vi "Configure Harmonic.vi"(0 "VISA resource name":refnum<visa-resource-name>, 1 "Enable Harmonic (F:Disable)":bool, 2 "Phase (0 Degree)":dbl, 5 "Output Channel (1: Channel 1)":i32(ring)=1 items=["Channel 1"=1, "Channel 2"=2], 7 "Order (2)":i32=2, 9 "Harmonic Type (0: Even)":i32(ring) items=["Even", "Odd", "All"], 11 "error in (no error)":errorcluster, 12 "Amplitude (1 Vpp)":dbl=1.0) -> (4 "VISA resource name out":refnum<visa-resource-name>, 15 "error out":errorcluster)   [LabVIEW 2015, in "SDG X Series.lvlib"]
doc: "Configures and enables harmonic output."
uses:
  <instrlib>/SDG X Series/SDG X Series.lvlib
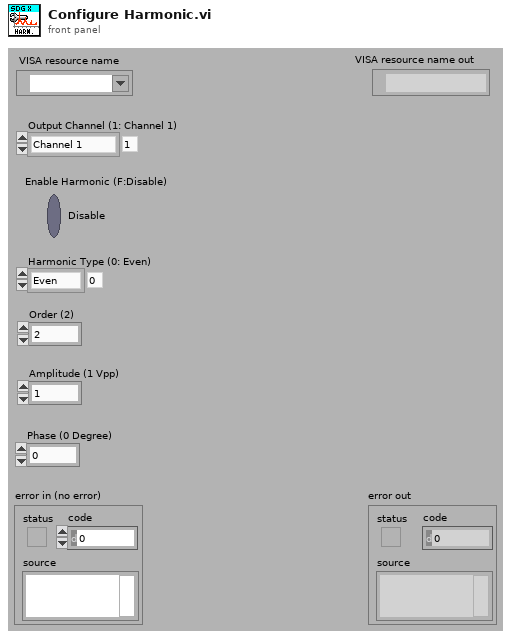
[diagram p1: front panel]
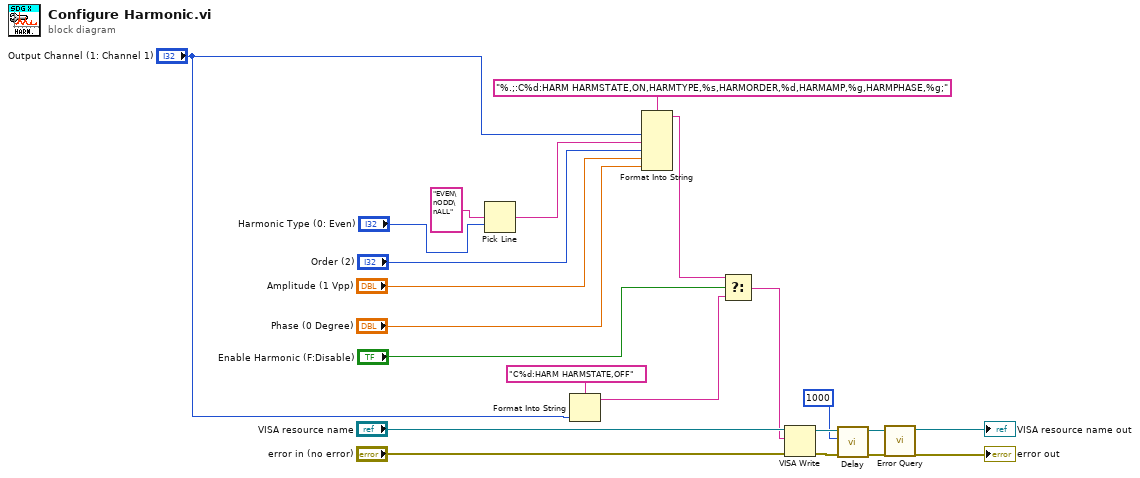
[diagram p0: block diagram]
diagram:
  n1 = Pick Line(multi-line string="EVEN\nODD\nALL", line index="Harmonic Type (0: Even)") -> (output string=w16:string)  [unwired: 1 out]
  n2 = Format Into String(format string="C%d:HARM HARMSTATE,OFF", "Output Channel (1: Channel 1)") -> (resulting string=w7:string)  [unwired: 2 in, 1 out]
  n3 = Format Into String(format string="%.;:C%d:HARM HARMSTATE,ON,HARMTYPE,%s,HARMORDER,%d,HARMAMP,%g,HARMPHASE,%g;", "Output Channel (1: Channel 1)", w16, "Order (2)", "Amplitude (1 Vpp)", "Phase (0 Degree)") -> (resulting string=w11:string)  [unwired: 2 in, 1 out]
  n4 = Select(t=w11, s="Enable Harmonic (F:Disable)", f=w7) -> (s? t:f=w10:string)
  n5 = VISA Write(VISA resource name="VISA resource name", write buffer=w10, error in (no error)="error in (no error)") -> (VISA resource name out=w3:refnum<visa-resource-name>, error out=w2:errorcluster)  [unwired: 1 out]
  n6 = call <instrlib>:"Delay.vi"("error in (no error)"=w2, "Delay Time (10)"=u32 1000, "VISA resource name"=w3) -> ("error out"=w5:errorcluster, "VISA resource name out"=w4:refnum<visa-resource-name>)  [unwired: 7 in]
  n7 = call <instrlib>:"Error Query.vi"("error in (no error)"=w5, "VISA resource name"=w4) -> ("error out"=→"error out":errorcluster, "VISA resource name out"=→"VISA resource name out":refnum<visa-resource-name>)  [unwired: 6 in, 2 out]
